vi "GDSString_SplitStrings_Array.vi"(0 "string":string, 1 "Max string length":i32=40) -> (14 "Array":string[](array[string]))   [LabVIEW 2020]
panel:
  out "Array 2":i32[](array[numeric])
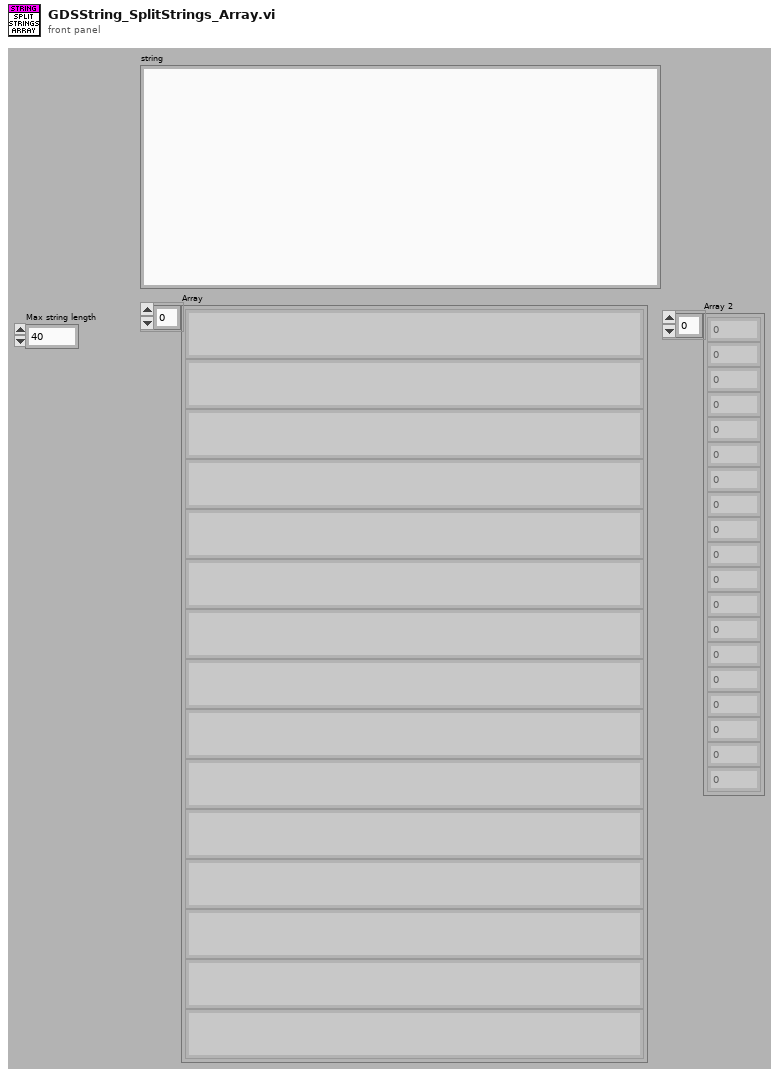
[diagram p1: front panel]
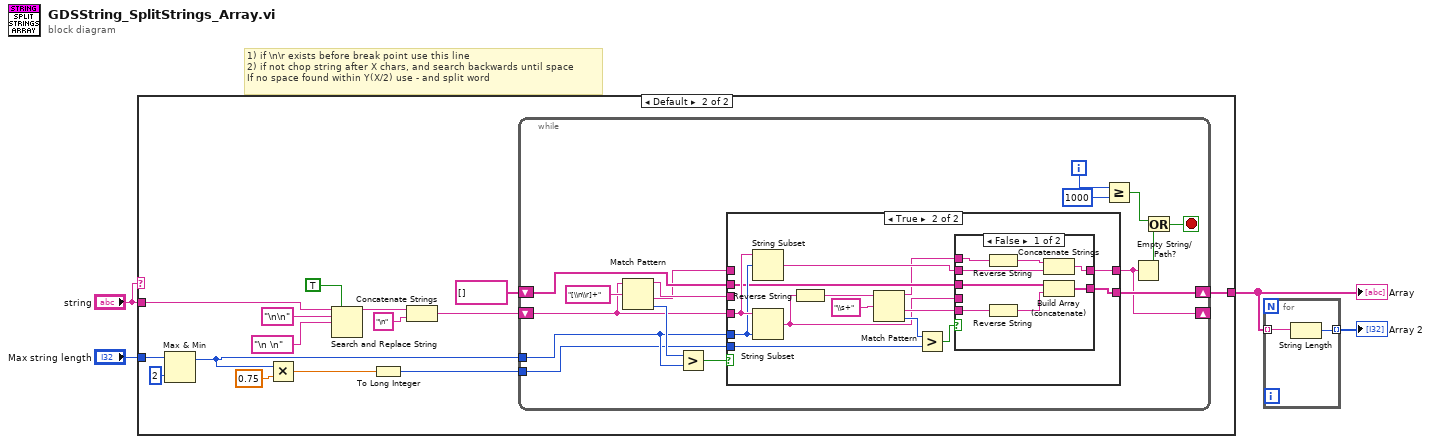
[diagram p0: block diagram]
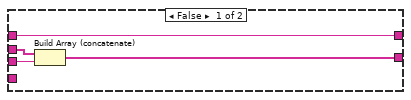
[diagram p3: hidden frame]
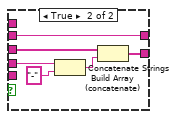
[diagram p4: hidden frame]
diagram:
  # "1) if \\n\\r exists before break point use this line\n2) if not chop string after X chars, and search backwards until space\nIf no space found within Y(X/2) use - and split word"
  n1 = case shown="Default" "string" {
    tunnel: "Max string length" -> [_ w7]
    tunnel: [_ w15] -> w3
    tunnel: "string" -> [_ w9]
    frame "" {
    }
    frame Default {
      n2 = Max & Min(x=w7, y=2) -> (max(x,y)=w5:i32)  [unwired: 1 out]
      n3 = Multiply(x=w5, y=0.75) -> (x*y=w17:dbl)
      n4 = Search and Replace String(replace all?=TRUE ("replace all? (F)"), input string=w9, search string="\n\n" ("string"), replace string="\n \n" ("string")) -> (result string=w8:string)  [unwired: 1 in, 6 out]
      n5 = To Long Integer(number=w17) -> (32bit integer=w16:i32)
      n6 = Concatenate Strings(w8, "\n" ("string")) -> (w13:string)
      n7 = while {
        shift-right: [w25] -> _
        shift-left: w13 -> [w28]
        shift-right: [w30] -> w15
        shift-left: string[] [] -> [w33]
        tunnel: w5 -> [w27]
        tunnel: w16 -> [w26]
        i -> [w24]
        stop <- w20 stop-if-true
        n8 = Match Pattern(string=w28, regular expression="[\\n\\r]+") -> (before substring=w31:string, after substring=w29:string, offset past match=w34:i32)  [unwired: 2 out]
        n9 = Greater?(x=w34, y=w27) -> (0:w32:bool)
        n10 = case shown="True" w32 {
          tunnel: w33 -> [w39 w44]
          tunnel: w31 -> [w38 _]
          tunnel: [w37 w43] -> w30
          tunnel: w29 -> [w36 _]
          tunnel: [w36 w45] -> w25
          tunnel: w28 -> [_ w48]
          tunnel: w27 -> [_ w47]
          tunnel: w26 -> [_ w50]
          frame False {
            n11 = Build Array (concatenate)(w39, w38) -> (w37:string[])
          }
          frame True {
            n12 = String Subset(string=w48, offset (0)=w47) -> (substring=w46:string)  [unwired: 1 out]
            n13 = String Subset(string=w48, length (rest)=w47) -> (substring=w40:string)  [unwired: 1 out]
            n14 = Reverse String(1:w40) -> (0:w53:string)
            n15 = Match Pattern(string=w53, regular expression="\\s+") -> (before substring=w42:string, after substring=w41:string, offset past match=w51:i32)  [unwired: 2 out]
            n16 = Greater?(x=w51, y=w50) -> (0:w49:bool)
            n17 = case shown="False" w49 {
              tunnel: w46 -> [w55 w67]
              tunnel: [w54 w67] -> w45
              tunnel: w44 -> [w61 w64]
              tunnel: [w60 w63] -> w43
              tunnel: w41 -> [w59 _]
              tunnel: w42 -> [w57 _]
              tunnel: w40 -> [_ w66]
              frame False {
                n18 = Reverse String(1:w57) -> (0:w56:string)
                n19 = Reverse String(1:w59) -> (0:w58:string)
                n20 = Concatenate Strings(w56, w55) -> (w54:string)
                n21 = Build Array (concatenate)(w61, w58) -> (w60:string[])
              }
              frame True {
                n22 = Concatenate Strings(w66, "-" ("string")) -> (w62:string)
                n23 = Build Array (concatenate)(w64, w62) -> (w63:string[])
              }
            }
          }
        }
        n24 = Greater Or Equal?(x=w24, y=1000) -> (x >= y?=w22:bool)
        n25 = Empty String/Path?(string/path=w25) -> (empty?=w21:bool)
        n26 = Or(x=w22, y=w21) -> (x .or. y?=w20:bool)
      }
    }
  }
  "Array" <- w3
  n27 = for {
    tunnel: w3 -> [w69] mode=indexing
    tunnel: [w68] -> w2 mode=indexing
    n28 = String Length(string=w69) -> (length=w68:i32)
  }
  "Array 2" <- w2
